vi "Connect via TLS.vi"(8 "error in":errorcluster, 10 "Certificates":T1, 11 "Connection Config":T2) -> (0 "error out":errorcluster, 2 "server certificate chain":cluster{"certificate":u8[]}[](array[cluster]), 3 "TCP Network Connection out":refnum<k5>)   [LabVIEW 2020, in "MQTT Client.lvclass"]
uses:
  MQTT Client.lvclass
  mqttTypedef/ConnectionConfig.ctl
  mqttTypedef/Certificates.ctl
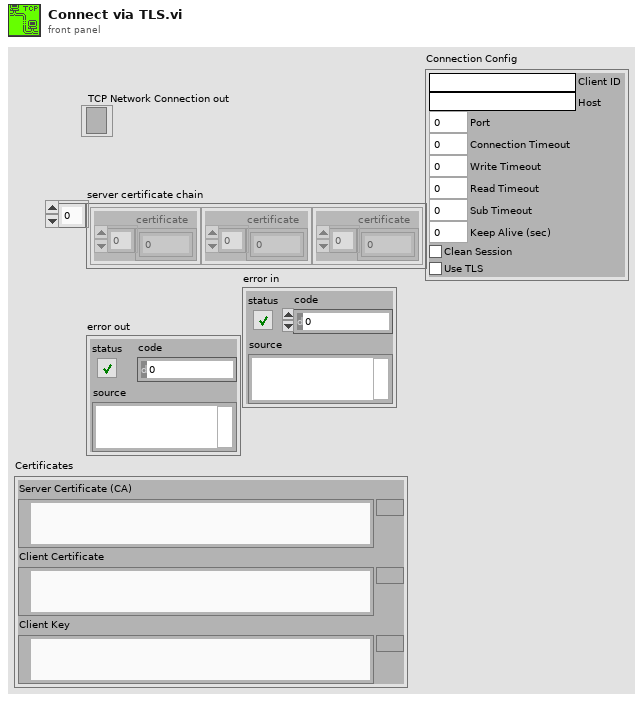
[diagram p1: front panel]
types:
  T1 = typedef "MQTT Client.lvclass/Certificates.ctl" = cluster{"Server Certificate (CA)":path, "Client Certificate":path, "Client Key":path}
  T2 = typedef "MQTT Client.lvclass/ConnectionConfig.ctl" = cluster{"Client ID":string, "Host":string, "Port":u16, "Connection Timeout":i32, "Write Timeout":i32, "Read Timeout":i32, "Sub Timeout":i32, "Keep Alive (sec)":u16, "Clean Session":bool, "Use TLS":bool}
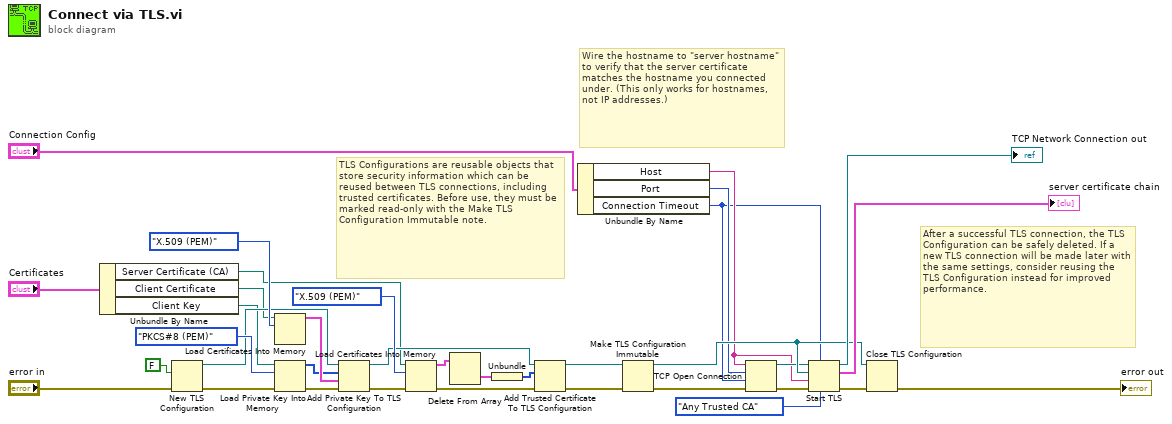
[diagram p0: block diagram]
diagram:
  # "Wire the hostname to \"server hostname\" to verify that the server certificate matches the hostname you connected under. (This only works for hostnames, not IP addresses.)"
  # "TLS Configurations are reusable objects that store security information which can be reused between TLS connections, including trusted certificates. Before use, they must be marked read-only with the Make TLS Configuration Immutable note."
  # "After a successful TLS connection, the TLS Configuration can be safely deleted. If a new TLS connection will be made later with the same settings, consider reusing the TLS Configuration instead for improved performance."
  n1 = Unbundle By Name("Certificates") -> ("Server Certificate (CA)"=w7:path, "Client Certificate"=w6:path, "Client Key"=w5:path)
  n2 = New TLS Configuration(8:"error in", 10:FALSE ("load OS trusted CAs?")) -> (0:w20:errorcluster, 3:w19:refnum<k36>)
  n3 = Load Certificates Into Memory(10:enum32{"X.509 (PEM)"}."X.509 (PEM)" ("format"), 11:w6) -> (3:w31:cluster{"certificate":u8[]}[])  [unwired: 1 in, 1 out]
  n4 = Load Private Key Into Memory(8:w20, 10:enum32{"PKCS#8 (PEM)", "PKCS#8 (DER)"}."PKCS#8 (PEM)" ("format"), 11:w5) -> (0:w21:errorcluster, 3:w22:u8[])  [unwired: 1 in]
  n5 = Add Private Key To TLS Configuration(8:w21, 9:w31, 10:w22, 11:w19) -> (0:w4:errorcluster, 3:w23:refnum<k36>)
  n6 = Load Certificates Into Memory(8:w4, 10:enum32{"X.509 (PEM)"}."X.509 (PEM)" ("format"), 11:w7) -> (0:w3:errorcluster, 3:w29:cluster{"certificate":u8[]}[])
  n7 = Delete From Array(array=w29) -> (deleted portion=w27:cluster{"certificate":u8[]})  [unwired: 2 in, 1 out]
  n8 = Unbundle(w27) -> ("certificate"=w28:u8[])
  n9 = Add Trusted Certificate To TLS Configuration(8:w3, 10:w28, 11:w23) -> (0:w25:errorcluster, 3:w24:refnum<k36>)
  n10 = Unbundle By Name("Connection Config") -> ("Host"=w9:string, "Port"=w2:u16, "Connection Timeout"=w1:i32)
  n11 = Make TLS Configuration Immutable(8:w25, 11:w24) -> (0:w12:errorcluster, 3:w16:refnum<k36>)
  n12 = TCP Open Connection(address=w9, remote port or service name=w2, timeout ms (60000)=w1, error in (no error)=w12) -> (connection ID=w13:refnum<k5>, error out=w14:errorcluster)  [unwired: 1 in]
  n13 = Start TLS(6:enum32{"Any Trusted CA", "None"}."Any Trusted CA" ("server certificate validation"), 7:w1, 8:w14, 9:w9, 10:w16, 11:w13) -> (0:w15:errorcluster, 2:→"server certificate chain":cluster{"certificate":u8[]}[], 3:→"TCP Network Connection out":refnum<k5>)
  n14 = Close TLS Configuration(8:w15, 11:w16) -> (0:→"error out":errorcluster)
